vi "Set Current Limit.vi"(8 "error in (no error)":errorcluster, 10 "Current Limit (I)":dbl, 11 "Keysight Power Supply in":refnum<class "Keysight Power Supply.lvclass">) -> (0 "error out":errorcluster, 3 "Keysight Power Supply out":refnum<class "Keysight Power Supply.lvclass">)   [LabVIEW 2017, in "Power Supply Driver.lvlib" / "Keysight Power Supply.lvclass"]
uses:
  Keysight Power Supply.lvclass
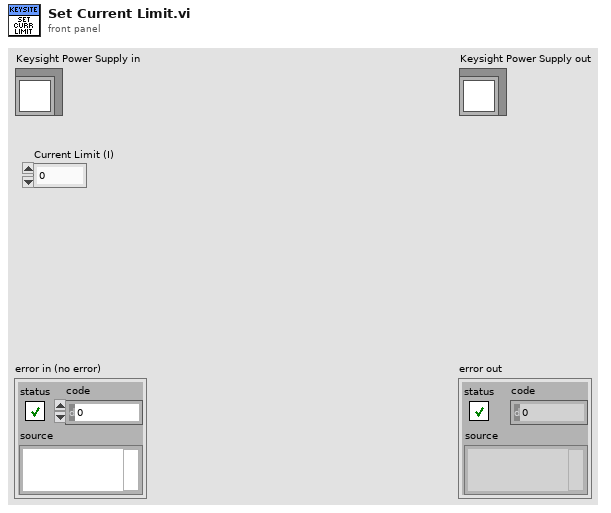
[diagram p1: front panel]
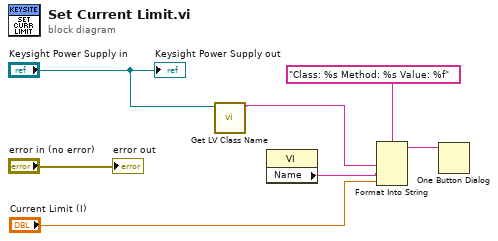
[diagram p0: block diagram]
diagram:
  n1 = call <vilib>:"Get LV Class Name.vi"("object"="Keysight Power Supply in") -> ("class name"=w5:string)  [unwired: 9 in, 1 out]
  n2 = property class="VI"() -> ("Name"=w4:string)  [unwired: 2 in, 2 out]
  n3 = Format Into String(format string="Class: %s Method: %s Value: %f", w5, w4, "Current Limit (I)") -> (resulting string=w3:string)  [unwired: 2 in, 1 out]
  n4 = One Button Dialog(message=w3) -> ()  [unwired: 1 in, 1 out]
  "error out" <- "error in (no error)"
  "Keysight Power Supply out" <- "Keysight Power Supply in"
